vi "scanWaveGen_deBullshit.vi"(6 "overScanBlanking":bool, 8 "singleDirScan":bool, 9 "numRoundingPts":u16, 10 "scanWaveForm":T2(ring), 11 "numPts":u16) -> (2 "blankingParams":T1, 3 "outWave":dbl[](array[numeric]))   [LabVIEW 2016]
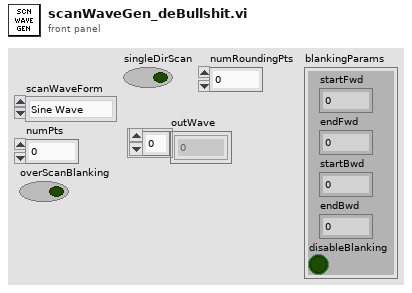
[diagram p1: front panel]
types:
  T1 = cluster{"startFwd":u16, "endFwd":u16, "startBwd":u16, "endBwd":u16, "disableBlanking":bool}
  T2 = enum16{"Sine Wave", "Triangle Wave", "Rounded Triangle"}
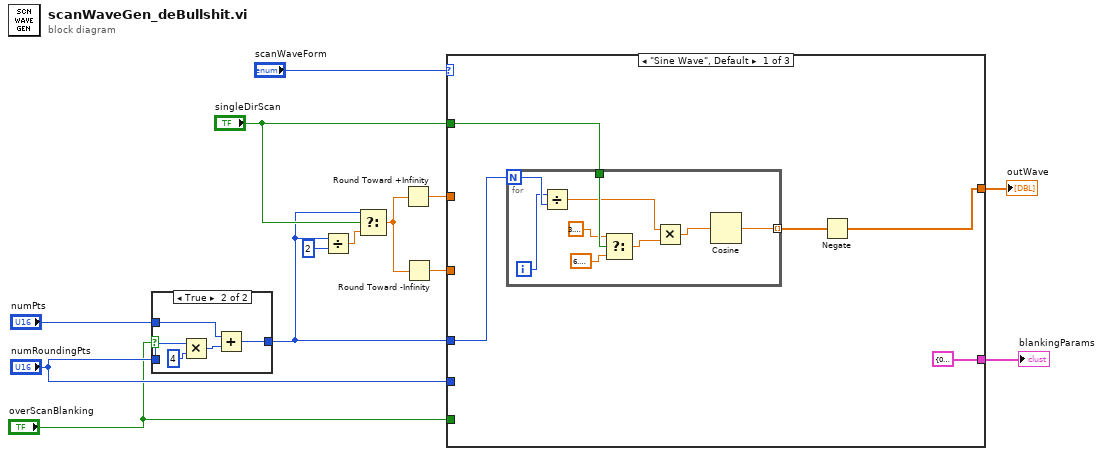
[diagram p0: block diagram]
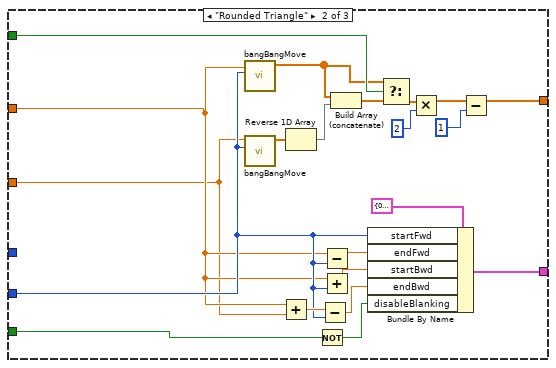
[diagram p3: hidden frame]
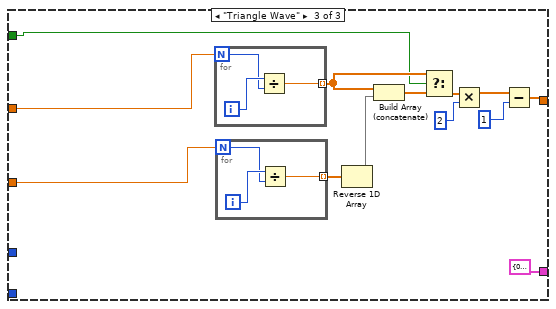
[diagram p4: hidden frame]
diagram:
  n1 = case shown="True" "overScanBlanking" {
    tunnel: "numRoundingPts" -> [_ w19]
    tunnel: "numPts" -> [w14 w16]
    tunnel: [w14 w15] -> w1
    frame False {
    }
    frame True {
      n2 = Multiply(x=w19, y=4) -> (x*y=w17:i32)
      n3 = Add(x=w16, y=w17) -> (x+y=w15:i32)
    }
  }
  n4 = Divide(x=w1, y=i16 2) -> (x/y=w6:dbl)
  n5 = Select(t=w1, s="singleDirScan", f=w6) -> (s? t:f=w7:dbl)
  n6 = Round Toward +Infinity(x=w7) -> (ceil(x): smallest int >= x=w3:dbl)
  n7 = Round Toward -Infinity(1:w7) -> (0:w2:dbl)
  n8 = case shown="\"Sine Wave\", Default" "scanWaveForm" {
    tunnel: "singleDirScan" -> [w24 w47 w56]
    tunnel: "numRoundingPts" -> [_ w42 _]
    tunnel: [w20 w50 w55] -> w13
    tunnel: "overScanBlanking" -> [_ w40 _]
    tunnel: [T1 {"startFwd"=0, "endFwd"=0, "startBwd"=0, "endBwd"=0, "disableBlanking"=TRUE} ("fastBlanking") w38 T1 {"startFwd"=0, "endFwd"=0, "startBwd"=0, "endBwd"=0, "disableBlanking"=TRUE} ("fastBlanking")] -> w9
    tunnel: w3 -> [_ w37 w66]
    tunnel: w2 -> [_ w36 w65]
    tunnel: w1 -> [w22 _ _]
    frame "Sine Wave", Default {
      n9 = for {
        N: w22 -> [w33]
        tunnel: w24 -> [w31]
        tunnel: [w25] -> w23 mode=indexing
        i -> [w32]
        n10 = Divide(x=w32, y=w33) -> (x/y=w27:dbl)
        n11 = Select(t=3.141592653589793, s=w31, f=6.283185307179586) -> (s? t:f=w28:dbl)
        n12 = Multiply(x=w27, y=w28) -> (x*y=w26:dbl)
        n13 = Cosine(x=w26) -> (cos(x)=w25:dbl)
      }
      n14 = Negate(x=w23) -> (-x=w20:dbl[])
    }
    frame "Rounded Triangle" {
      n15 = call "bangBangMove.vi"("numRoundingPts"=w42, "numPts"=w37) -> ("roundedHalfTriangle"=w35:dbl[])  [unwired: 9 in]
      n16 = call "bangBangMove.vi"("numRoundingPts"=w42, "numPts"=w36) -> ("roundedHalfTriangle"=w54:dbl[])  [unwired: 9 in]
      n17 = Add(x=w37, y=w36) -> (x+y=w43:dbl)
      n18 = Reverse 1D Array(array=w54) -> (reversed array=w34:dbl[])
      n19 = Not(x=w40) -> (.not. x?=w39:bool)
      n20 = Subtract(x=w43, y=w42) -> (x-y=w41:dbl)
      n21 = Subtract(x=w37, y=w42) -> (x-y=w45:dbl)
      n22 = Add(x=w37, y=w42) -> (x+y=w44:dbl)
      n23 = Build Array (concatenate)(w35, w34) -> (w53:dbl[])
      n24 = Bundle By Name(cluster=T1 {"startFwd"=0, "endFwd"=0, "startBwd"=0, "endBwd"=0, "disableBlanking"=FALSE} ("fastBlanking"), "startFwd"=w42, "endFwd"=w45, "startBwd"=w44, "endBwd"=w41, "disableBlanking"=w39) -> (w38:T1)
      n25 = Select(t=w35, s=w47, f=w53) -> (s? t:f=w48:dbl[])
      n26 = Multiply(x=w48, y=2) -> (x*y=w52:dbl[])
      n27 = Subtract(x=w52, y=1) -> (x-y=w50:dbl[])
    }
    frame "Triangle Wave" {
      n28 = for {
        N: w66 -> [w72]
        tunnel: [w71] -> w57 mode=indexing
        i -> [w73]
        n29 = Divide(x=w73, y=w72) -> (x/y=w71:dbl)
      }
      n30 = for {
        N: w65 -> [w69]
        tunnel: [w68] -> w64 mode=indexing
        i -> [w70]
        n31 = Divide(x=w70, y=w69) -> (x/y=w68:dbl)
      }
      n32 = Reverse 1D Array(array=w64) -> (reversed array=w58:dbl[])
      n33 = Build Array (concatenate)(w57, w58) -> (w59:dbl[])
      n34 = Select(t=w57, s=w56, f=w59) -> (s? t:f=w63:dbl[])
      n35 = Multiply(x=w63, y=2) -> (x*y=w60:dbl[])
      n36 = Subtract(x=w60, y=1) -> (x-y=w55:dbl[])
    }
  }
  "outWave" <- w13
  "blankingParams" <- w9
